vi "main.vi"() -> ()   [LabVIEW 2018]
panel:
  in  "子面板2":bool
  in  "子面板1":bool
  in  "退出":bool caption="停止"
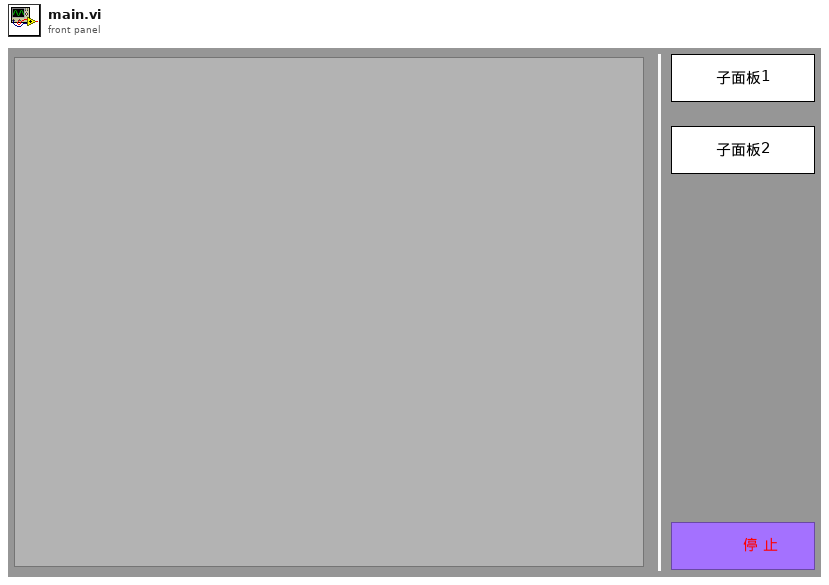
[diagram p1: front panel]
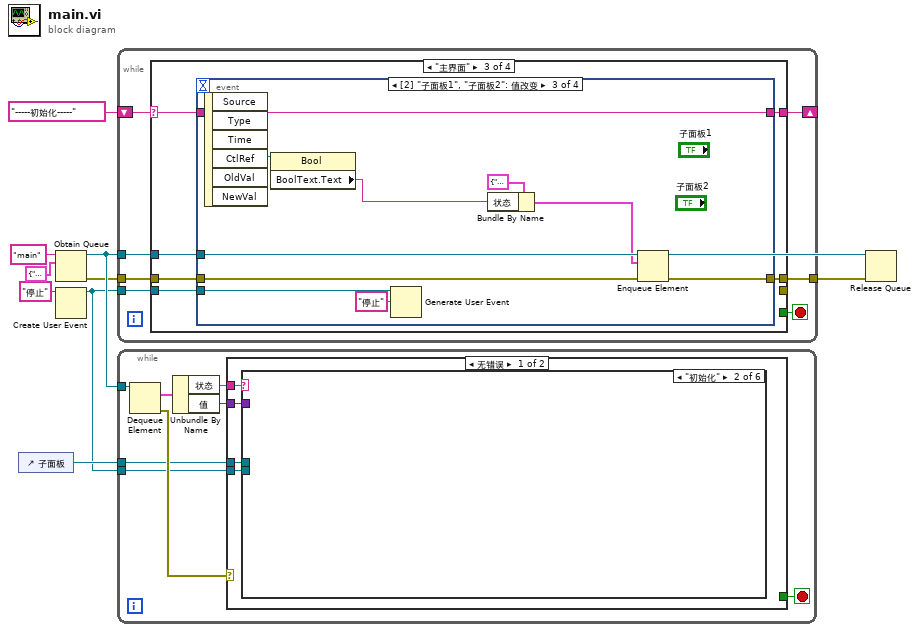
[diagram p0: block diagram]
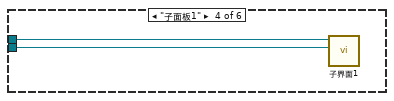
[diagram p4: hidden frame]
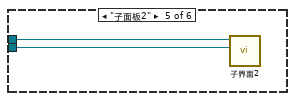
[diagram p5: hidden frame]
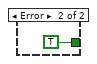
[diagram p7: hidden frame]
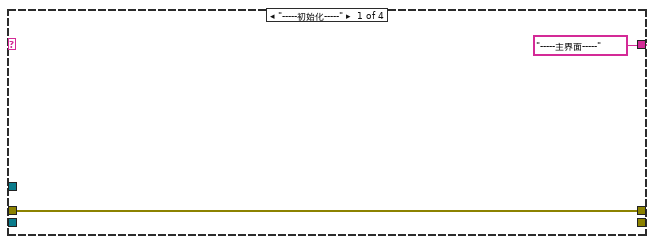
[diagram p8: hidden frame]
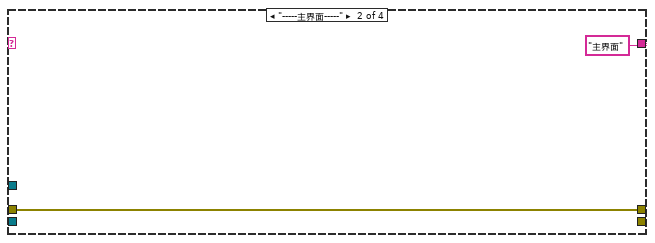
[diagram p9: hidden frame]
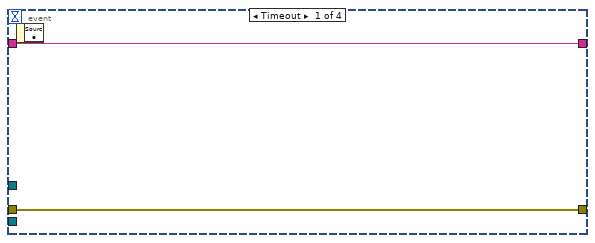
[diagram p10: hidden frame]
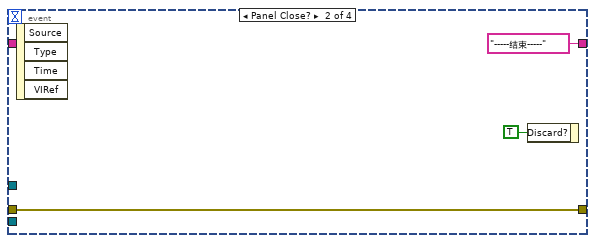
[diagram p11: hidden frame]
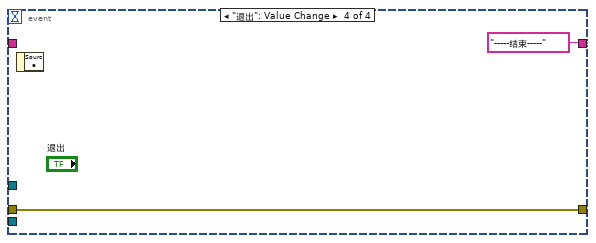
[diagram p12: hidden frame]
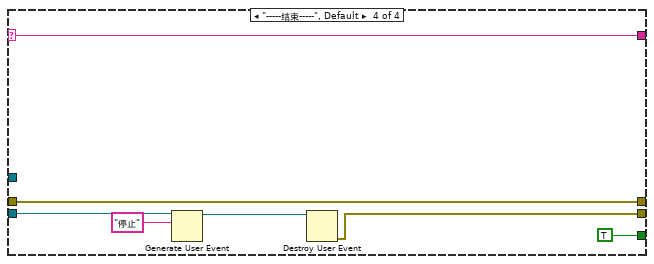
[diagram p13: hidden frame]
diagram:
  n1 = control-ref of="子面板"() -> (w3:refnum<vi>)
  n2 = Obtain Queue(name (unnamed)="main" ("名称（未命名）"), element data type=cluster{"状态":string, "值":variant} {"状态"="", "值"=variant} ("队列元素")) -> (queue out=w9:refnum<queue>, error out=w7:errorcluster)  [unwired: 3 in, 1 out]
  n3 = Create User Event(user event datatype="停止" ("停止")) -> (user event=w1:refnum<user-event>)  [unwired: 1 in, 1 out]
  n4 = while {
    tunnel: w9 -> [w16]
    shift-right: [w15] -> _
    shift-left: "-----初始化-----" -> [w14]
    tunnel: w7 -> [w12]
    tunnel: [w11] -> w6
    tunnel: w1 -> [w10]
    stop <- w13 stop-if-true
    n5 = case shown="\"主界面\"" w14 {
      selector: w14 -> [_ _ w22 w49]
      tunnel: w16 -> [_ _ w26 _]
      tunnel: w12 -> [w17 w19 w25 w50]
      tunnel: [w17 w19 w24 w50] -> w11
      tunnel: ["-----主界面-----" "主界面" w23 w49] -> w15
      tunnel: [_ _ _ TRUE] -> w13
      tunnel: w10 -> [_ _ w21 w46]
      tunnel: [_ _ _ w44] -> _
      frame "-----初始化-----" {
      }
      frame "-----主界面-----" {
      }
      frame "主界面" {
        n6 = event shown="[2] \"子面板1\", \"子面板2\": 值改变" {
          selector: _ -> [_ _ _ _]
          dyn-events: _ -> [_ _ _ _]
          timeout: _ -> [_ _ _ _]
          tunnel: w26 -> [_ _ w40 _]
          tunnel: w25 -> [w27 w30 w39 w43]
          tunnel: [w27 w30 w38 w43] -> w24
          tunnel: [w28 "-----结束-----" w41 "-----结束-----"] -> w23
          tunnel: w22 -> [w28 _ w41 _]
          tunnel: w21 -> [_ _ w32 _]
          event Timeout {
            n7 = event-data() -> ()  [unwired: 1 in, 1 out]
          }
          event Panel Close? {
            n8 = event-data() -> ()  [unwired: 1 in, 4 out]
            n9 = event-data("Discard?"=TRUE ("放弃？")) -> ()  [unwired: 1 in, 1 out]
          }
          event "子面板1", "子面板2": Value Change {
            n10 = event-data() -> ("CtlRef"=w37:refnum<vi>)  [unwired: 1 in, 5 out]
            n11 = property class="Bool"(reference=w37) -> ("BoolText.Text"=w35:string)  [unwired: 1 in, 2 out]
            n12 = Generate User Event(user event=w32, event data cluster="停止" ("事件数据")) -> ()  [unwired: 2 in, 2 out]
            n13 = Bundle By Name(cluster=cluster{"状态":string, "值":variant} {"状态"="", "值"=variant} ("元素"), "状态"=w35) -> (w34:cluster{"状态":string, "值":variant})
            n14 = Enqueue Element(queue=w40, element=w34, error in (no error)=w39) -> (error out=w38:errorcluster)  [unwired: 1 in, 2 out]
          }
          event "退出": Value Change {
            n15 = event-data() -> ()  [unwired: 1 in, 1 out]
          }
        }
      }
      frame "-----结束-----", Default {
        n16 = Generate User Event(user event=w46, event data cluster="停止" ("事件数据")) -> (user event out=w45:refnum<user-event>)  [unwired: 2 in, 1 out]
        n17 = Destroy User Event(user event=w45) -> (error out=w44:errorcluster)  [unwired: 1 in]
      }
    }
  }
  n18 = while {
    tunnel: w9 -> [w58]
    tunnel: w3 -> [w52]
    tunnel: w1 -> [w51]
    stop <- w56 stop-if-true
    n19 = Dequeue Element(queue=w58) -> (element=w55:cluster{"状态":string, "值":variant}, error out=w57:errorcluster)  [unwired: 2 in, 2 out]
    n20 = Unbundle By Name(w55) -> ("状态"=w54:string, "值"=w53:variant)
    n21 = case shown="无错误" w57 {
      tunnel: [_ TRUE] -> w56
      tunnel: w54 -> [w62 _]
      tunnel: w53 -> [w61 _]
      tunnel: w52 -> [w60 _]
      tunnel: w51 -> [w59 _]
      frame No Error {
        n22 = case shown="\"初始化\"" w62 {
          tunnel: w61 -> [_ _ _ _ _ _]
          tunnel: w60 -> [_ _ _ w64 w66 _]
          tunnel: w59 -> [_ _ _ w63 w65 _]
          frame "假", Default {
          }
          frame "初始化" {
          }
          frame "-----子面板-----" {
          }
          frame "子面板1" {
            n23 = call "子界面1.vi"("用户事件输出"=w63, "子面板"=w64) -> ()  [unwired: 10 in]
          }
          frame "子面板2" {
            n24 = call "子界面2.vi"("用户事件输出"=w65, "子面板"=w66) -> ()  [unwired: 10 in]
          }
          frame "结束" {
          }
        }
      }
      frame Error {
      }
    }
  }
  n25 = Release Queue(queue=w9, error in (no error)=w6) -> ()  [unwired: 1 in, 3 out]
